vi "Read Analog Data.vi"(8 "error in (no error)":errorcluster, 11 "Analog Input Waveform Data Msg in":refnum<class "Analog Input Waveform Data Msg.lvclass">) -> (0 "error out":errorcluster, 2 "Analog Data":waveform(dbl)[](array[waveform]), 3 "Analog Input Waveform Data Msg out":refnum<class "Analog Input Waveform Data Msg.lvclass">)   [LabVIEW 2024, in "DAQmx Actor Interface.lvlib" / "Analog Input Waveform Data Msg.lvclass"]
uses:
  Analog Input Waveform Data Msg.lvclass
  Analog Input Waveform Data Msg.lvclass/Analog Input Waveform Data Msg.ctl
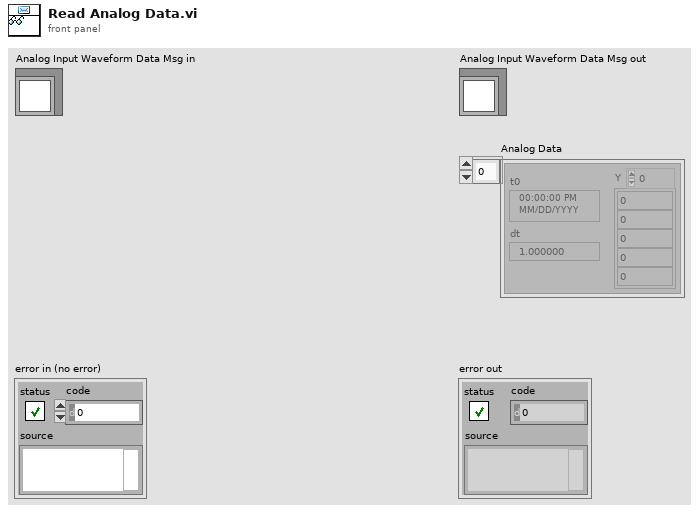
[diagram p1: front panel]
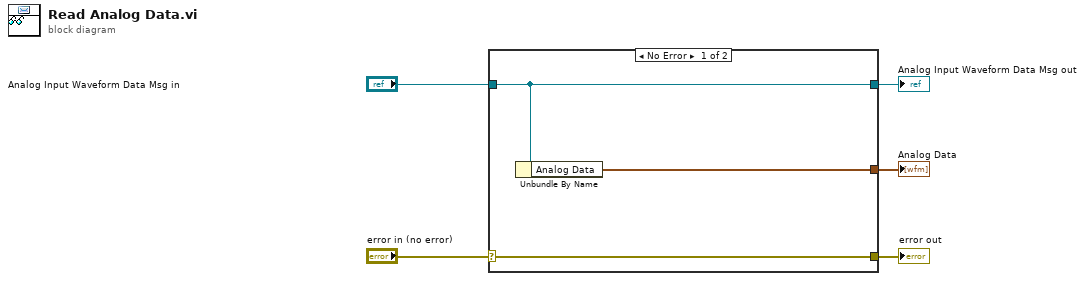
[diagram p0: block diagram]
diagram:
  n1 = case shown="No Error" "error in (no error)" {
    selector: "error in (no error)" -> [w8 w9]
    tunnel: [w8 w9] -> w4
    tunnel: [w7 w10] -> w2
    tunnel: "Analog Input Waveform Data Msg in" -> [w7 w10]
    tunnel: [w6 _] -> w1
    frame No Error {
      n2 = Unbundle By Name(w7) -> ("Analog Data"=w6:waveform(dbl)[])
    }
    frame Error {
    }
  }
  "error out" <- w4
  "Analog Input Waveform Data Msg out" <- w2
  "Analog Data" <- w1
